vi "picoquant_plot_histogram.vi"(8 "error in (no error)":errorcluster, 9 "initialize_histogram?":bool, 10 "data":T1, 11 "hydraharp in":refnum<class "hydraharp.lvclass">) -> (0 "error out":errorcluster, 2 "histogram":cluster{"Axis":dbl[], "Histogram":i32[]}, 3 "hydraharp out":refnum<class "hydraharp.lvclass">)   [LabVIEW 2015, in "hydraharp.lvclass"]
uses:
  hydraharp.lvclass
  Picoquant_generic/picoquant_data_tdef.ctl
  hydraharp.lvclass/hydraharp.ctl
  <vilib>/Analysis/NI_AALPro.lvlib
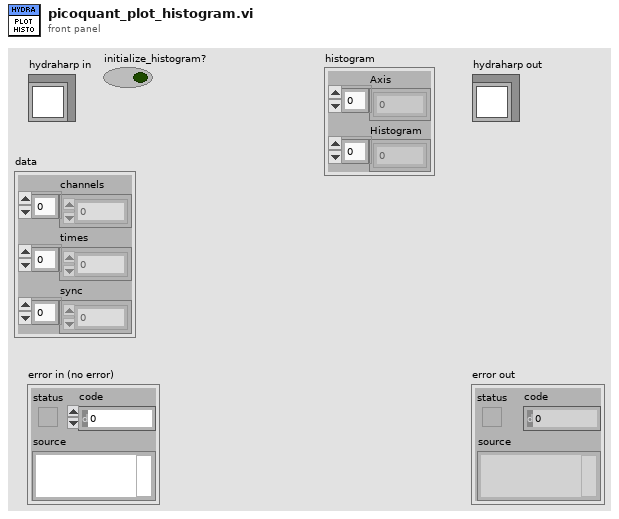
[diagram p1: front panel]
types:
  T1 = typedef "picoquant_data_tdef.ctl" = cluster{"channels":u8[], "times":u64[], "sync":u64[]}
  T2 = cluster{"lower":dbl, "upper":dbl, "inclusion":enum32{"lower", "upper", "both", "neither"}}
  T3 = typedef "hydra_histo_bins_tdef.ctl" = cluster{"lower":dbl, "upper":dbl, "inclusion":enum32{"lower", "upper", "both", "neither"}}[]
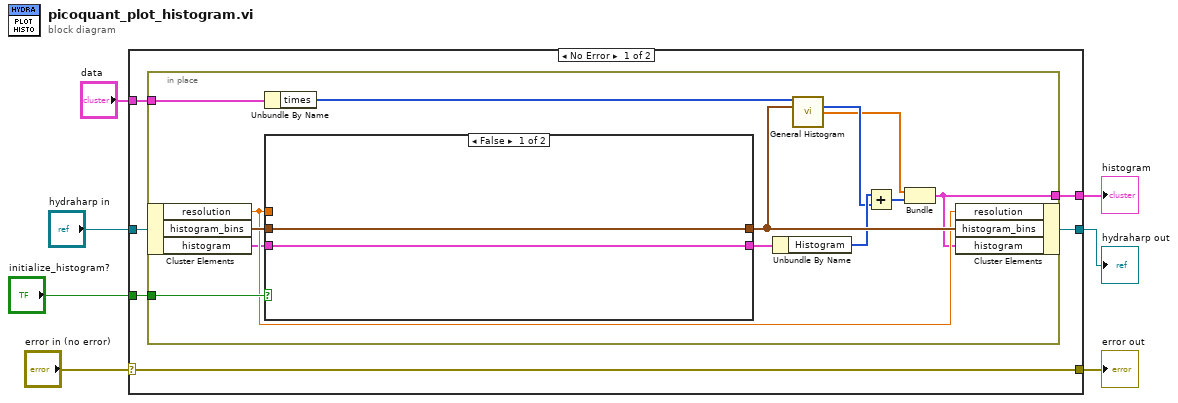
[diagram p0: block diagram]
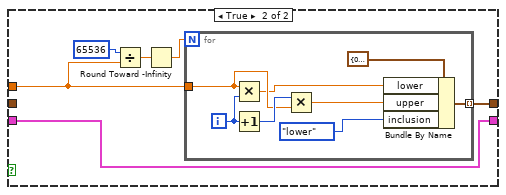
[diagram p2: hidden frame]
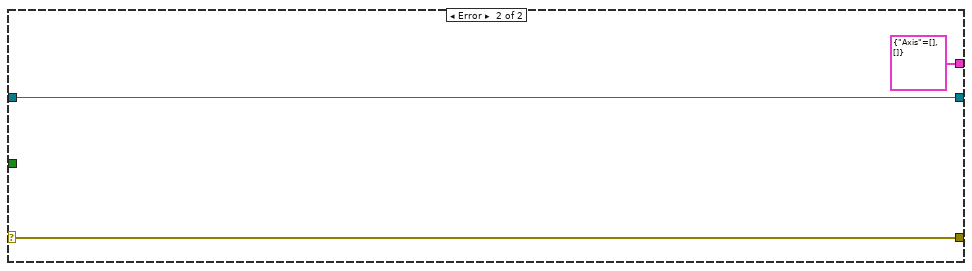
[diagram p3: hidden frame]
diagram:
  n1 = case shown="No Error" "error in (no error)" {
    selector: "error in (no error)" -> [w9 w45]
    tunnel: "hydraharp in" -> [w13 w44]
    tunnel: "initialize_histogram?" -> [w12 _]
    tunnel: "data" -> [w11 _]
    tunnel: [w10 cluster{"Axis":dbl[], i32[]} {"Axis"=[], []}] -> w3
    tunnel: [w9 w45] -> w2
    tunnel: [w8 w44] -> w1
    frame No Error {
      n2 = in-place {
        in-place-border: w12 -> [w26]
        in-place-border: w11 -> [w25]
        in-place-border: [w14] -> w10
        n3 = in-place-cluster #1(w13) -> ("resolution"=w21:dbl, "histogram_bins"=w23:T3, "histogram"=w20:cluster{"Axis":dbl[], "Histogram":i32[]})
        n4 = Unbundle By Name(w25) -> ("times"=w24:u64[])
        n5 = case shown="False" w26 {
          tunnel: w21 -> [_ w31]
          tunnel: [w28 w30] -> w22
          tunnel: w23 -> [w28 _]
          tunnel: w20 -> [w27 w29]
          tunnel: [w27 w29] -> w19
          frame False {
          }
          frame True {
            n6 = Divide(x=65536, y=w31) -> (x/y=w33:dbl)
            n7 = Round Toward -Infinity(1:w33) -> (0:w32:dbl)
            n8 = for {
              N: w32 -> [_]
              tunnel: w31 -> [w40]
              tunnel: [w35] -> w30 mode=indexing
              i -> [w41]
              n9 = Multiply(x=w40, y=w41) -> (x*y=w38:dbl)
              n10 = Increment(x=w41) -> (x+1=w42:i32)
              n11 = Multiply(x=w42, y=w40) -> (x*y=w37:dbl)
              n12 = Bundle By Name(cluster=T2 {"lower"=0.0, "upper"=0.0, "inclusion"=enum."lower"} ("element"), "lower"=w38, "upper"=w37, "inclusion"=enum32{"lower", "upper", "both", "neither"}."lower") -> (w35:T2)
            }
          }
        }
        n13 = Unbundle By Name(w19) -> ("Histogram"=w18:i32[])
        n14 = call <vilib>:"General Histogram.vi"("X"=w24, "Bins"=w22) -> ("Histogram"=w17:i32[], "Axis"=w15:dbl[])  [unwired: 9 in, 3 out]
        n15 = Add(x=w18, y=w17) -> (x+y=w16:i32[])
        n16 = Bundle("Axis"=w15, w16) -> (w14:cluster{"Axis":dbl[], i32[]})  [unwired: 1 in]
        n17 = in-place-cluster #1("resolution"=w21, "histogram_bins"=w22, "histogram"=w14) -> (w8:refnum<class "hydraharp.lvclass">)
      }
    }
    frame Error {
    }
  }
  "error out" <- w2
  "hydraharp out" <- w1
  "histogram" <- w3
